vi "HConfig (SubVI).vi"(9 "Names":string[](array[string]), 10 "DAQmx Selector":cluster{"On":bool, "physical channels":tag}[](array[cluster])=[{"On"=TRUE, "physical channels"="cDAQ1Mod1/ai0"}, {"On"=TRUE, "physical channels"="cDAQ1Mod1/ai1"}], 11 "Keyphasor":tag="cDAQ1Mod3/ai0") -> (2 "Channels and Names":string[][](array[string]), 3 "String":string)   [LabVIEW 2012]
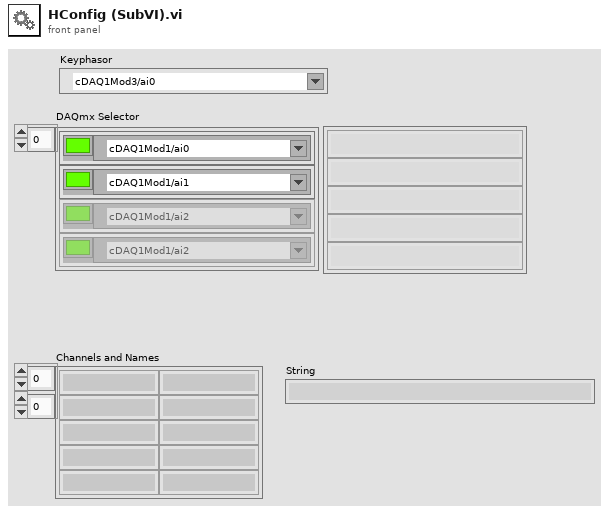
[diagram p1: front panel]
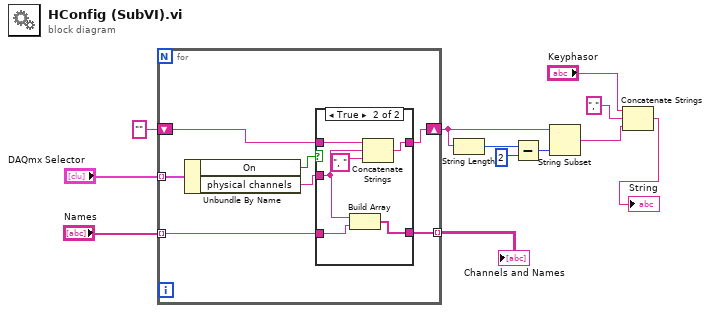
[diagram p0: block diagram]
diagram:
  n1 = for {
    tunnel: "DAQmx Selector" -> [w19] mode=indexing
    shift-right: [w16] -> w5
    shift-left: "" -> [w15]
    tunnel: "Names" -> [w14] mode=indexing
    tunnel: [w13] -> w1 mode=indexing
    n2 = Unbundle By Name(w19) -> ("On"=w17:bool, "physical channels"=w18:tag)
    n3 = case shown="True" w17 {
      tunnel: w18 -> [_ w23]
      tunnel: [w20 w26] -> w16
      tunnel: w15 -> [w20 w25]
      tunnel: w14 -> [_ w22]
      tunnel: [_ w21] -> w13
      frame False {
      }
      frame True {
        n4 = Build Array(w23, w22) -> (w21:string[])
        n5 = Concatenate Strings(w25, w23, ", ") -> (w26:string)
      }
    }
  }
  "Channels and Names" <- w1
  n6 = String Length(string=w5) -> (length=w6:i32)
  n7 = Subtract(x=w6, y=2 ("x")) -> (x-y=w7:i32)
  n8 = String Subset(string=w5, length (rest)=w7) -> (substring=w11:string)  [unwired: 1 in]
  n9 = Concatenate Strings("Keyphasor", "," ("string"), w11) -> (→"String":string)
